vi "Wind Check.vi"(8 "에러 입력(에러 없음)":errorcluster, 10 "강풍":dbl, 11 "현재 풍속":dbl) -> (0 "에러 출력":errorcluster, 1 "풍속 경고?":bool, 2 "풍속 경소 메시지":string caption="풍속 경고 메시지")   [LabVIEW 2010]
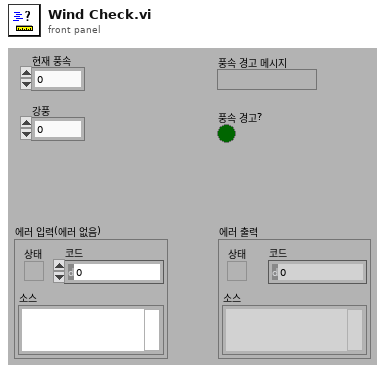
[diagram p1: front panel]
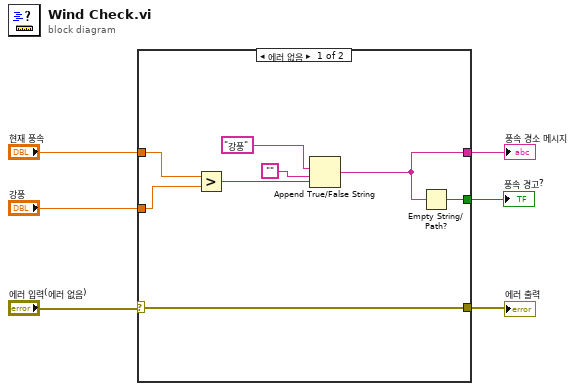
[diagram p0: block diagram]
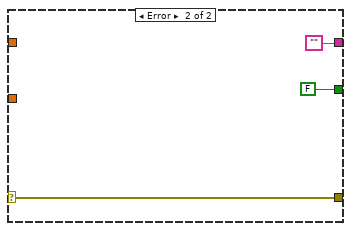
[diagram p2: hidden frame]
diagram:
  n1 = case shown="에러 없음" "에러 입력(에러 없음)" {
    selector: "에러 입력(에러 없음)" -> [w13 w17]
    tunnel: "현재 풍속" -> [w8 _]
    tunnel: "강풍" -> [w9 _]
    tunnel: [w7 ""] -> w4
    tunnel: [w14 FALSE] -> w3
    tunnel: [w13 w17] -> w1
    frame No Error {
      n2 = Greater?(x=w8, y=w9) -> (0:w10:bool)
      n3 = Append True/False String(1:w10, 2:"", 3:"강풍") -> (0:w7:string)  [unwired: 1 out]
      n4 = Empty String/Path?(string/path=w7) -> (empty?=w14:bool)
    }
    frame Error {
    }
  }
  "풍속 경소 메시지" <- w4
  "풍속 경고?" <- w3
  "에러 출력" <- w1
